vi "Autonomous Independent.vi"   [LabVIEW 2015]
doc: "This VI is called when autonomous begins, and will automatically be terminated when autonomous ends. You can carry out timed or sensor driven robot movement independently without needing to return to the caller."
uses:
  <vilib>/Rock Robotics/WPI/Solenoid/WPI_SolenoidValue.ctl
  <vilib>/Rock Robotics/WPI/Utilities/WPI_GetSetVariantRefNum.vi
  <vilib>/Rock Robotics/Network Tables/NT Read String.vi
  Robot Global Data.vi
  <vilib>/Rock Robotics/WPI/Solenoid/WPI_SolenoidSetEnum.vi
  <vilib>/Rock Robotics/Network Tables/NT Write Numeric Array.vi
panel:
  # "Be sure to right-click and choose Data Operations>>Make Current Value default if you want to save the array values with the VI"
types:
  T1 = typedef "WPI_JoystickDevRef.ctl" = cluster{"Device":T2}
  T2 = typedef "WPI_JoystickDeviceEnum.ctl" = enum16{"USB 0", "USB 1", "USB 2", "USB 3", "USB 4", "USB 5"}
  T3 = typedef "WPI_SolenoidValue.ctl" = enum16{"Off", "On", "Forward", "Reverse"}
  T4 = typedef "WPI_RobotDriveDevRef.ctl" = cluster{"DevStatus":errorcluster, "Motors[]":T5[], "Square Inputs":bool, "Max Output":dbl}
  T5 = typedef "WPI_MotorControlDeviceRef.ctl" = cluster{"DeviceStatus":errorcluster, "Type":T6, "PWM":cluster{"PWM Channel":T7, "DeadBand":T8}, "CAN":cluster{"Device Number":u8, "Control Mode":T9, "Semaphore":T10, "Max Vout":dbl, "TalonSRX Control Mode":T11}, "Invert":bool}
  T6 = typedef "WPI_MotorControlType.ctl" = enum16{"PWM", "CAN", "CANTalonSRX"}
  T7 = typedef "FPGA_DIOPWMChannel.ctl" = enum8{"PWM 0", "PWM 1", "PWM 2", "PWM 3", "PWM 4", "PWM 5", "PWM 6", "PWM 7", "PWM 8", "PWM 9", "PWM MXP 0", "PWM MXP 1", "PWM MXP 2", "PWM MXP 3", "PWM MXP 4", "PWM MXP 5", "PWM MXP 6", "PWM MXP 7", "PWM MXP 8", "PWM MXP 9", "Invalid"}
  T8 = typedef "WPI_PWMDeadband.ctl" = cluster{"Name":string, "maxPositivePwm":i32, "minPositivePwm":i32, "centerPwm":i32, "maxNegativePwm":i32, "minNegativePwm":i32, "angularRange":u16}
  T9 = typedef "WPI_CANJaguar_ControlMode.ctl" = enum8{"Percent VBus", "Current", "Speed", "Position", "Voltage"}
  T10 = typedef "Semaphore RefNum" = refnum<k1>
  T11 = typedef "WPI_CANTalonSRX_APIControlMode.ctl" = enum8{"Percent VBus", "Speed", "Position", "Slave", "Unchanged / Invalid", "Voltage Compensation", "Current", "Motion Profile"}
  T12 = typedef "WPI_SolenoidDevRef.ctl" = cluster{"DevStatus":errorcluster, "Pneumatics Control Module":u8, "Forward Solenoid Channel":T13, "Reverse Solenoid Channel":T13}
  T13 = typedef "WPI_SolenoidChannel.ctl" = enum8{"Solenoid 0", "Solenoid 1", "Solenoid 2", "Solenoid 3", "Solenoid 4", "Solenoid 5", "Solenoid 6", "Solenoid 7", "Invalid"}
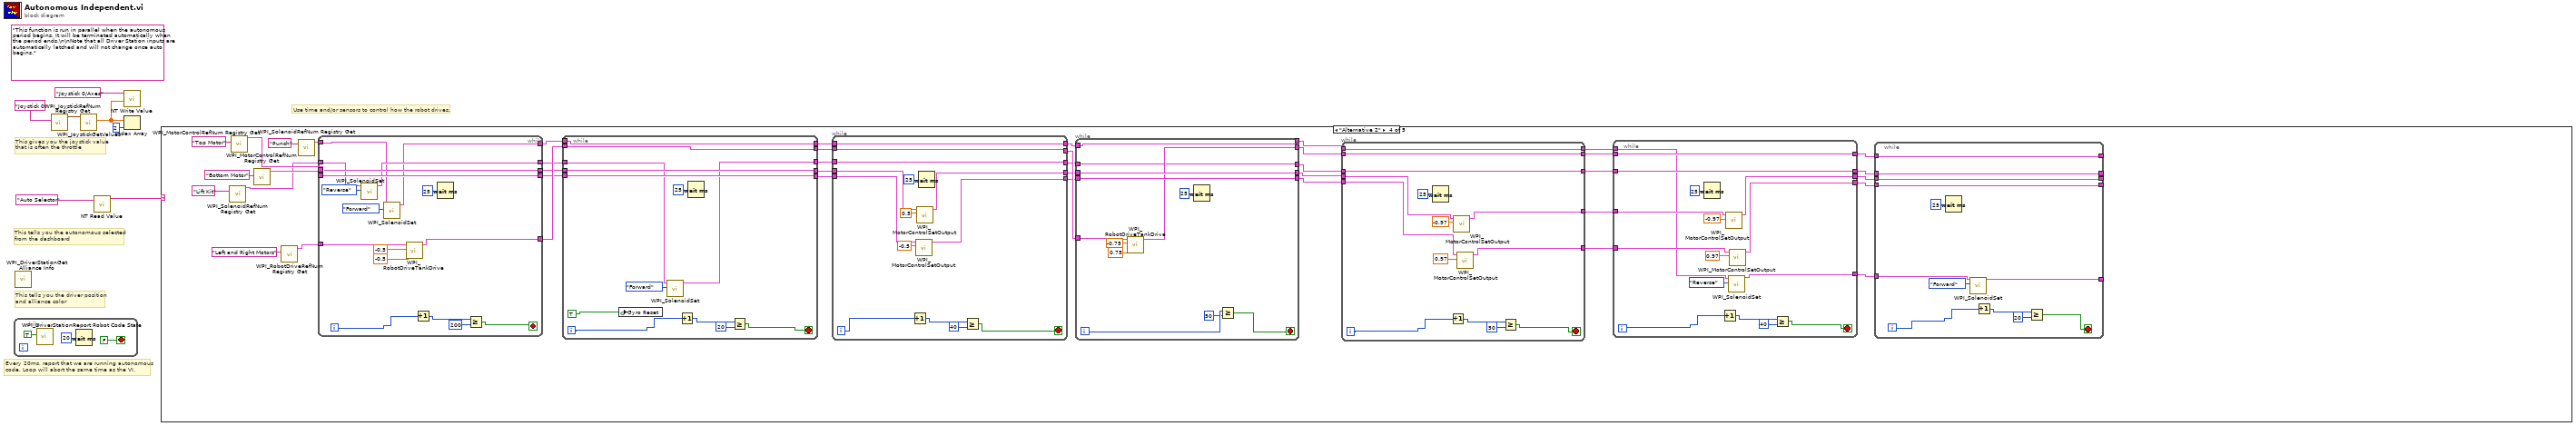
[diagram p0: block diagram]
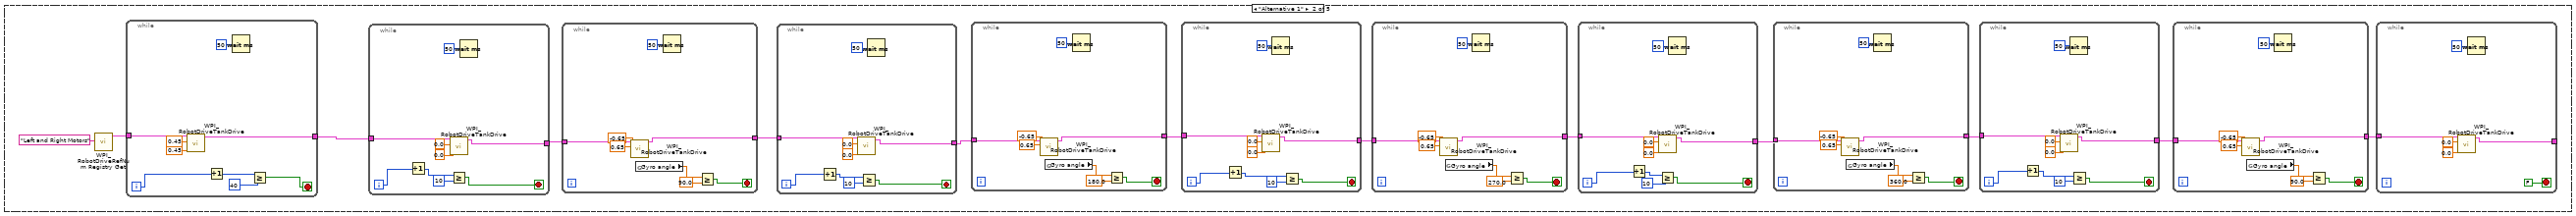
[diagram p3: hidden frame]
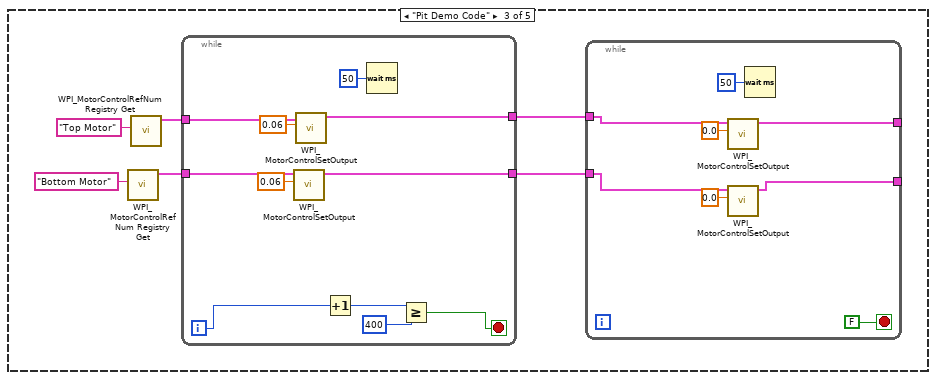
[diagram p4: hidden frame]
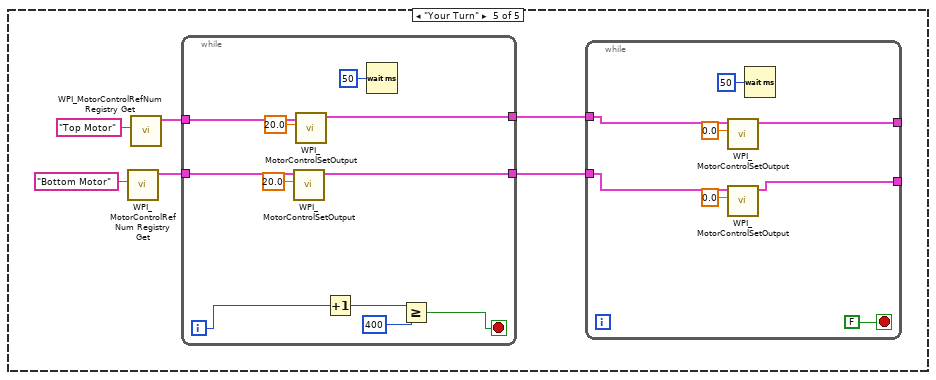
[diagram p5: hidden frame]
diagram:
  (unwired) "This function is run in parallel when the autonomous period begins. It will be terminated automatically when the period ends.\n\nNote that all Driver Station inputs are automatically latched and will not change once auto begins."
  # "This tells you the autonomous selected\nfrom the dashboard"
  # "Every 20ms, report that we are running autonomous\ncode. Loop will abort the same time as the VI."
  # "This gives you the joystick value\nthat is often the throttle"
  # "Use time and/or sensors to control how the robot drives."
  # "This tells you the driver position\nand alliance color"
  n1 = while {
    stop <- FALSE stop-if-true
    n2 = call <vilib>:"WPI_DriverStationReport Robot Code State.vi"("Autonomous"=TRUE) -> ()  [unwired: 10 in, 1 out]
    n3 = Wait (ms)(milliseconds to wait=u32 20) -> ()  [unwired: 1 out]
  }
  n4 = call <vilib>:"WPI_DriverStationGet Alliance Info.vi"() -> ()  [unwired: 12 out]
  n5 = call <vilib>:"WPI_JoystickRefNum Registry Get.vi"("refnum name"="Joystick 0") -> ("JoystickDevRef"=w6:T1)  [unwired: 1 in, 9 out]
  n6 = call <vilib>:"WPI_JoystickGetValues.vi"("JoystickDevRef"=w6) -> ("Axes"=w2:dbl[])  [unwired: 6 in, 4 out]
  n7 = call-poly <vilib>:"NT Read Value.vi"("Name"="Auto Selector") -> ("String"=w3:string)  [unwired: 9 in, 1 out]
  n8 = call-poly <vilib>:"NT Write Value.vi"("Numeric Array"=w2, "Name"="Joystick 0/Axes") -> ()  [unwired: 9 in, 1 out]
  n9 = Index Array(array=w2, index=2) -> ()  [unwired: 1 out]
  n10 = case shown="\"Alternative 2\"" w3 {
    frame Default {
      # "You can put your main auto here, or you can right-click on the case and make any\nother frame be the default case."
      # "This is the frame that will execute if no selection is made, or if it is not recognized"
    }
    frame "Alternative 1" {
      n11 = call <vilib>:"WPI_RobotDriveRefNum Registry Get.vi"("refnum name"="Left and Right Motors") -> ("RobotDriveDevRef"=w23:T4)  [unwired: 9 in, 1 out]
      n12 = while {
        tunnel: w23 -> [w118]
        tunnel: [w117] -> w22
        i -> [w120]
        stop <- w121 stop-if-true
        n13 = call <vilib>:"WPI_RobotDriveTankDrive.vi"("Right axis value"=0.45, "Left axis value"=0.45, "RobotDriveDevRef"=w118) -> ("RobotDriveDevRef"=w117:T4)  [unwired: 6 in, 2 out]
        n14 = Increment(x=w120) -> (x+1=w122:i32)
        n15 = Wait (ms)(milliseconds to wait=u32 50) -> ()  [unwired: 1 out]
        n16 = Greater Or Equal?(x=w122, y=40) -> (x >= y?=w121:bool)
      }
      n17 = while {
        tunnel: w22 -> [w113]
        tunnel: [w110] -> w20
        i -> [w109]
        stop <- w106 stop-if-true
        n18 = Increment(x=w109) -> (x+1=w108:i32)
        n19 = call <vilib>:"WPI_RobotDriveTankDrive.vi"("Right axis value"=0.0, "Left axis value"=0.0, "RobotDriveDevRef"=w113) -> ("RobotDriveDevRef"=w110:T4)  [unwired: 6 in, 2 out]
        n20 = Greater Or Equal?(x=w108, y=10) -> (x >= y?=w106:bool)
        n21 = Wait (ms)(milliseconds to wait=u32 50) -> ()  [unwired: 1 out]
      }
      n22 = while {
        tunnel: w20 -> [w105]
        tunnel: [w98] -> w19
        stop <- w100 stop-if-true
        n23 = call <vilib>:"WPI_RobotDriveTankDrive.vi"("Right axis value"=-0.65, "Left axis value"=0.65, "RobotDriveDevRef"=w105) -> ("RobotDriveDevRef"=w98:T4)  [unwired: 6 in, 2 out]
        n24 = global read "Robot Global Data.vi" "Gyro angle"() -> (w101:dbl)
        n25 = Wait (ms)(milliseconds to wait=u32 50) -> ()  [unwired: 1 out]
        n26 = Greater Or Equal?(x=w101, y=90.0) -> (x >= y?=w100:bool)
      }
      n27 = while {
        tunnel: w19 -> [w96]
        tunnel: [w93] -> w18
        i -> [w92]
        stop <- w89 stop-if-true
        n28 = Increment(x=w92) -> (x+1=w91:i32)
        n29 = call <vilib>:"WPI_RobotDriveTankDrive.vi"("Right axis value"=0.0, "Left axis value"=0.0, "RobotDriveDevRef"=w96) -> ("RobotDriveDevRef"=w93:T4)  [unwired: 6 in, 2 out]
        n30 = Greater Or Equal?(x=w91, y=10) -> (x >= y?=w89:bool)
        n31 = Wait (ms)(milliseconds to wait=u32 50) -> ()  [unwired: 1 out]
      }
      n32 = while {
        tunnel: w18 -> [w88]
        tunnel: [w81] -> w17
        stop <- w83 stop-if-true
        n33 = call <vilib>:"WPI_RobotDriveTankDrive.vi"("Right axis value"=-0.65, "Left axis value"=0.65, "RobotDriveDevRef"=w88) -> ("RobotDriveDevRef"=w81:T4)  [unwired: 6 in, 2 out]
        n34 = global read "Robot Global Data.vi" "Gyro angle"() -> (w84:dbl)
        n35 = Wait (ms)(milliseconds to wait=u32 50) -> ()  [unwired: 1 out]
        n36 = Greater Or Equal?(x=w84, y=180.0) -> (x >= y?=w83:bool)
      }
      n37 = while {
        tunnel: w17 -> [w79]
        tunnel: [w76] -> w16
        i -> [w75]
        stop <- w72 stop-if-true
        n38 = Increment(x=w75) -> (x+1=w74:i32)
        n39 = call <vilib>:"WPI_RobotDriveTankDrive.vi"("Right axis value"=0.0, "Left axis value"=0.0, "RobotDriveDevRef"=w79) -> ("RobotDriveDevRef"=w76:T4)  [unwired: 6 in, 2 out]
        n40 = Wait (ms)(milliseconds to wait=u32 50) -> ()  [unwired: 1 out]
        n41 = Greater Or Equal?(x=w74, y=10) -> (x >= y?=w72:bool)
      }
      n42 = while {
        tunnel: w16 -> [w71]
        tunnel: [w64] -> w15
        stop <- w66 stop-if-true
        n43 = call <vilib>:"WPI_RobotDriveTankDrive.vi"("Right axis value"=-0.65, "Left axis value"=0.65, "RobotDriveDevRef"=w71) -> ("RobotDriveDevRef"=w64:T4)  [unwired: 6 in, 2 out]
        n44 = global read "Robot Global Data.vi" "Gyro angle"() -> (w67:dbl)
        n45 = Wait (ms)(milliseconds to wait=u32 50) -> ()  [unwired: 1 out]
        n46 = Greater Or Equal?(x=w67, y=270.0) -> (x >= y?=w66:bool)
      }
      n47 = while {
        tunnel: w15 -> [w62]
        tunnel: [w59] -> w14
        i -> [w58]
        stop <- w55 stop-if-true
        n48 = Increment(x=w58) -> (x+1=w57:i32)
        n49 = call <vilib>:"WPI_RobotDriveTankDrive.vi"("Right axis value"=0.0, "Left axis value"=0.0, "RobotDriveDevRef"=w62) -> ("RobotDriveDevRef"=w59:T4)  [unwired: 6 in, 2 out]
        n50 = Greater Or Equal?(x=w57, y=10) -> (x >= y?=w55:bool)
        n51 = Wait (ms)(milliseconds to wait=u32 50) -> ()  [unwired: 1 out]
      }
      n52 = while {
        tunnel: w14 -> [w54]
        tunnel: [w47] -> w13
        stop <- w49 stop-if-true
        n53 = call <vilib>:"WPI_RobotDriveTankDrive.vi"("Right axis value"=-0.65, "Left axis value"=0.65, "RobotDriveDevRef"=w54) -> ("RobotDriveDevRef"=w47:T4)  [unwired: 6 in, 2 out]
        n54 = global read "Robot Global Data.vi" "Gyro angle"() -> (w50:dbl)
        n55 = Wait (ms)(milliseconds to wait=u32 50) -> ()  [unwired: 1 out]
        n56 = Greater Or Equal?(x=w50, y=360.0) -> (x >= y?=w49:bool)
      }
      n57 = while {
        tunnel: w13 -> [w45]
        tunnel: [w42] -> w12
        i -> [w41]
        stop <- w38 stop-if-true
        n58 = Increment(x=w41) -> (x+1=w40:i32)
        n59 = call <vilib>:"WPI_RobotDriveTankDrive.vi"("Right axis value"=0.0, "Left axis value"=0.0, "RobotDriveDevRef"=w45) -> ("RobotDriveDevRef"=w42:T4)  [unwired: 6 in, 2 out]
        n60 = Wait (ms)(milliseconds to wait=u32 50) -> ()  [unwired: 1 out]
        n61 = Greater Or Equal?(x=w40, y=10) -> (x >= y?=w38:bool)
      }
      n62 = while {
        tunnel: w12 -> [w37]
        tunnel: [w30] -> w11
        stop <- w32 stop-if-true
        n63 = call <vilib>:"WPI_RobotDriveTankDrive.vi"("Right axis value"=-0.65, "Left axis value"=0.65, "RobotDriveDevRef"=w37) -> ("RobotDriveDevRef"=w30:T4)  [unwired: 6 in, 2 out]
        n64 = global read "Robot Global Data.vi" "Gyro angle"() -> (w33:dbl)
        n65 = Wait (ms)(milliseconds to wait=u32 50) -> ()  [unwired: 1 out]
        n66 = Greater Or Equal?(x=w33, y=90.0) -> (x >= y?=w32:bool)
      }
      n67 = while {
        tunnel: w11 -> [w27]
        tunnel: [w24] -> _
        stop <- FALSE stop-if-true
        n68 = call <vilib>:"WPI_RobotDriveTankDrive.vi"("Right axis value"=0.0, "Left axis value"=0.0, "RobotDriveDevRef"=w27) -> ("RobotDriveDevRef"=w24:T4)  [unwired: 6 in, 2 out]
        n69 = Wait (ms)(milliseconds to wait=u32 50) -> ()  [unwired: 1 out]
      }
    }
    frame "Pit Demo Code" {
      n70 = call <vilib>:"WPI_MotorControlRefNum Registry Get.vi"("refnum name"="Bottom Motor") -> ("MotorControlDevRef"=w129:T5)  [unwired: 9 in, 1 out]
      n71 = call <vilib>:"WPI_MotorControlRefNum Registry Get.vi"("refnum name"="Top Motor") -> ("MotorControlDevRef"=w128:T5)  [unwired: 9 in, 1 out]
      n72 = while {
        tunnel: w129 -> [w148]
        tunnel: w128 -> [w147]
        tunnel: [w141] -> w125
        tunnel: [w140] -> w124
        i -> [w143]
        stop <- w144 stop-if-true
        n73 = call <vilib>:"WPI_MotorControlSetOutput.vi"("Output"=0.06, "MotorControlDevRef"=w148) -> ("MotorControlDevRef"=w140:T5)  [unwired: 7 in, 2 out]
        n74 = call <vilib>:"WPI_MotorControlSetOutput.vi"("Output"=0.06, "MotorControlDevRef"=w147) -> ("MotorControlDevRef"=w141:T5)  [unwired: 7 in, 2 out]
        n75 = Increment(x=w143) -> (x+1=w145:i32)
        n76 = Wait (ms)(milliseconds to wait=u32 50) -> ()  [unwired: 1 out]
        n77 = Greater Or Equal?(x=w145, y=400) -> (x >= y?=w144:bool)
      }
      n78 = while {
        tunnel: w125 -> [w135]
        tunnel: w124 -> [w133]
        tunnel: [w134] -> _
        tunnel: [w132] -> _
        stop <- FALSE stop-if-true
        n79 = call <vilib>:"WPI_MotorControlSetOutput.vi"("Output"=0.0, "MotorControlDevRef"=w135) -> ("MotorControlDevRef"=w134:T5)  [unwired: 7 in, 2 out]
        n80 = call <vilib>:"WPI_MotorControlSetOutput.vi"("Output"=0.0, "MotorControlDevRef"=w133) -> ("MotorControlDevRef"=w132:T5)  [unwired: 7 in, 2 out]
        n81 = Wait (ms)(milliseconds to wait=u32 50) -> ()  [unwired: 1 out]
      }
    }
    frame "Alternative 2" {
      n82 = call <vilib>:"WPI_SolenoidRefNum Registry Get.vi"("refnum name"="Lift Kit") -> ("SolenoidDevRef"=w174:T12)  [unwired: 9 in, 1 out]
      n83 = call <vilib>:"WPI_MotorControlRefNum Registry Get.vi"("refnum name"="Top Motor") -> ("MotorControlDevRef"=w181:T5)  [unwired: 9 in, 1 out]
      n84 = call <vilib>:"WPI_MotorControlRefNum Registry Get.vi"("refnum name"="Bottom Motor") -> ("MotorControlDevRef"=w179:T5)  [unwired: 9 in, 1 out]
      n85 = call <vilib>:"WPI_RobotDriveRefNum Registry Get.vi"("refnum name"="Left and Right Motors") -> ("RobotDriveDevRef"=w185:T4)  [unwired: 9 in, 1 out]
      n86 = call <vilib>:"WPI_SolenoidRefNum Registry Get.vi"("refnum name"="Punch") -> ("SolenoidDevRef"=w171:T12)  [unwired: 9 in, 1 out]
      n87 = while {
        tunnel: w185 -> [w286]
        tunnel: [w279] -> w182
        tunnel: w181 -> [w277]
        tunnel: [w277] -> w180
        tunnel: w179 -> [w276]
        tunnel: [w276] -> w178
        tunnel: w174 -> [w275]
        tunnel: [w274] -> w173
        tunnel: [w270] -> w170
        tunnel: w171 -> [w271]
        i -> [w280]
        stop <- w281 stop-if-true
        n88 = call-poly <vilib>:"WPI_SolenoidSet.vi"("Value"=WPI_SolenoidValue."Reverse", "SolenoidDevRef"=w275) -> ("SolenoidDevRef"=w274:T12)  [unwired: 8 in, 1 out]
        n89 = call-poly <vilib>:"WPI_SolenoidSet.vi"("Value"=WPI_SolenoidValue."Forward", "SolenoidDevRef"=w271) -> ("SolenoidDevRef"=w270:T12)  [unwired: 8 in, 1 out]
        n90 = call <vilib>:"WPI_RobotDriveTankDrive.vi"("Right axis value"=-0.5, "Left axis value"=-0.5, "RobotDriveDevRef"=w286) -> ("RobotDriveDevRef"=w279:T4)  [unwired: 6 in, 2 out]
        n91 = Increment(x=w280) -> (x+1=w283:i32)
        n92 = Wait (ms)(milliseconds to wait=u32 25) -> ()  [unwired: 1 out]
        n93 = Greater Or Equal?(x=w283, y=200) -> (x >= y?=w281:bool)
      }
      n94 = while {
        tunnel: [w227] -> w158
        tunnel: w182 -> [w227]
        tunnel: [w220] -> w154
        tunnel: w180 -> [w220]
        tunnel: [w219] -> w153
        tunnel: w178 -> [w219]
        tunnel: w173 -> [w217]
        tunnel: [w216] -> w152
        tunnel: w170 -> [w215]
        tunnel: [w215] -> w156
        i -> [w222]
        stop <- w223 stop-if-true
        n95 = global write "Robot Global Data.vi" "Gyro Reset"(TRUE) -> ()
        n96 = call-poly <vilib>:"WPI_SolenoidSet.vi"("Value"=WPI_SolenoidValue."Forward", "SolenoidDevRef"=w217) -> ("SolenoidDevRef"=w216:T12)  [unwired: 8 in, 1 out]
        n97 = Increment(x=w222) -> (x+1=w224:i32)
        n98 = Wait (ms)(milliseconds to wait=u32 25) -> ()  [unwired: 1 out]
        n99 = Greater Or Equal?(x=w224, y=20) -> (x >= y?=w223:bool)
      }
      n100 = while {
        tunnel: [w202] -> w157
        tunnel: w158 -> [w202]
        tunnel: [w201] -> w155
        tunnel: w156 -> [w201]
        tunnel: w154 -> [w200]
        tunnel: w153 -> [w199]
        tunnel: [w196] -> w151
        tunnel: w152 -> [w196]
        tunnel: [w195] -> w150
        tunnel: [w194] -> w149
        i -> [w190]
        stop <- w189 stop-if-true
        n101 = Increment(x=w190) -> (x+1=w192:i32)
        n102 = call <vilib>:"WPI_MotorControlSetOutput.vi"("Output"=-0.5, "MotorControlDevRef"=w199) -> ("MotorControlDevRef"=w194:T5)  [unwired: 7 in, 2 out]
        n103 = call <vilib>:"WPI_MotorControlSetOutput.vi"("Output"=0.5, "MotorControlDevRef"=w200) -> ("MotorControlDevRef"=w195:T5)  [unwired: 7 in, 2 out]
        n104 = Wait (ms)(milliseconds to wait=u32 25) -> ()  [unwired: 1 out]
        n105 = Greater Or Equal?(x=w192, y=40) -> (x >= y?=w189:bool)
      }
      n106 = while {
        tunnel: w157 -> [w269]
        tunnel: w150 -> [w265]
        tunnel: [w265] -> w160
        tunnel: [w264] -> w159
        tunnel: w149 -> [w264]
        tunnel: [w263] -> w162
        tunnel: [w262] -> w161
        tunnel: w151 -> [w262]
        tunnel: [w261] -> w163
        tunnel: w155 -> [w261]
        i -> [w260]
        stop <- w259 stop-if-true
        n107 = call <vilib>:"WPI_RobotDriveTankDrive.vi"("Right axis value"=0.75, "Left axis value"=-0.75, "RobotDriveDevRef"=w269) -> ("RobotDriveDevRef"=w263:T4)  [unwired: 6 in, 2 out]
        n108 = Wait (ms)(milliseconds to wait=u32 25) -> ()  [unwired: 1 out]
        n109 = Greater Or Equal?(x=w260, y=50) -> (x >= y?=w259:bool)
      }
      n110 = while {
        tunnel: [w250] -> w184
        tunnel: [w249] -> w183
        tunnel: w160 -> [w248]
        tunnel: w159 -> [w247]
        tunnel: [w246] -> w177
        tunnel: w162 -> [w246]
        tunnel: [w245] -> w172
        tunnel: w161 -> [w245]
        tunnel: w163 -> [w244]
        tunnel: [w244] -> w169
        i -> [w251]
        stop <- w252 stop-if-true
        n111 = Wait (ms)(milliseconds to wait=u32 25) -> ()  [unwired: 1 out]
        n112 = Increment(x=w251) -> (x+1=w254:i32)
        n113 = call <vilib>:"WPI_MotorControlSetOutput.vi"("Output"=-0.97, "MotorControlDevRef"=w248) -> ("MotorControlDevRef"=w250:T5)  [unwired: 7 in, 2 out]
        n114 = call <vilib>:"WPI_MotorControlSetOutput.vi"("Output"=0.97, "MotorControlDevRef"=w247) -> ("MotorControlDevRef"=w249:T5)  [unwired: 7 in, 2 out]
        n115 = Greater Or Equal?(x=w254, y=50) -> (x >= y?=w252:bool)
      }
      n116 = while {
        tunnel: w184 -> [w236]
        tunnel: w183 -> [w235]
        tunnel: [w233] -> w164
        tunnel: w177 -> [w233]
        tunnel: [w232] -> w165
        tunnel: w172 -> [w232]
        tunnel: w169 -> [w231]
        tunnel: [w230] -> w168
        tunnel: [w229] -> w166
        tunnel: [w228] -> w167
        i -> [w237]
        stop <- w238 stop-if-true
        n117 = Wait (ms)(milliseconds to wait=u32 25) -> ()  [unwired: 1 out]
        n118 = Increment(x=w237) -> (x+1=w240:i32)
        n119 = call <vilib>:"WPI_MotorControlSetOutput.vi"("Output"=-0.97, "MotorControlDevRef"=w236) -> ("MotorControlDevRef"=w229:T5)  [unwired: 7 in, 2 out]
        n120 = call-poly <vilib>:"WPI_SolenoidSet.vi"("Value"=WPI_SolenoidValue."Reverse", "SolenoidDevRef"=w231) -> ("SolenoidDevRef"=w230:T12)  [unwired: 8 in, 1 out]
        n121 = call <vilib>:"WPI_MotorControlSetOutput.vi"("Output"=0.97, "MotorControlDevRef"=w235) -> ("MotorControlDevRef"=w228:T5)  [unwired: 7 in, 2 out]
        n122 = Greater Or Equal?(x=w240, y=40) -> (x >= y?=w238:bool)
      }
      n123 = while {
        tunnel: w168 -> [w212]
        tunnel: w167 -> [w211]
        tunnel: w166 -> [w208]
        tunnel: w165 -> [w209]
        tunnel: w164 -> [w210]
        tunnel: [w211] -> _
        tunnel: [w210] -> _
        tunnel: [w209] -> _
        tunnel: [w208] -> _
        tunnel: [w207] -> _
        i -> [w203]
        stop <- w204 stop-if-true
        n124 = Wait (ms)(milliseconds to wait=u32 25) -> ()  [unwired: 1 out]
        n125 = call-poly <vilib>:"WPI_SolenoidSet.vi"("Value"=WPI_SolenoidValue."Forward", "SolenoidDevRef"=w212) -> ("SolenoidDevRef"=w207:T12)  [unwired: 8 in, 1 out]
        n126 = Increment(x=w203) -> (x+1=w205:i32)
        n127 = Greater Or Equal?(x=w205, y=20) -> (x >= y?=w204:bool)
      }
    }
    frame "Your Turn" {
      n128 = call <vilib>:"WPI_MotorControlRefNum Registry Get.vi"("refnum name"="Bottom Motor") -> ("MotorControlDevRef"=w292:T5)  [unwired: 9 in, 1 out]
      n129 = call <vilib>:"WPI_MotorControlRefNum Registry Get.vi"("refnum name"="Top Motor") -> ("MotorControlDevRef"=w291:T5)  [unwired: 9 in, 1 out]
      n130 = while {
        tunnel: w292 -> [w311]
        tunnel: w291 -> [w310]
        tunnel: [w304] -> w288
        tunnel: [w303] -> w287
        i -> [w306]
        stop <- w307 stop-if-true
        n131 = call <vilib>:"WPI_MotorControlSetOutput.vi"("Output"=20.0, "MotorControlDevRef"=w311) -> ("MotorControlDevRef"=w303:T5)  [unwired: 7 in, 2 out]
        n132 = call <vilib>:"WPI_MotorControlSetOutput.vi"("Output"=20.0, "MotorControlDevRef"=w310) -> ("MotorControlDevRef"=w304:T5)  [unwired: 7 in, 2 out]
        n133 = Increment(x=w306) -> (x+1=w308:i32)
        n134 = Wait (ms)(milliseconds to wait=u32 50) -> ()  [unwired: 1 out]
        n135 = Greater Or Equal?(x=w308, y=400) -> (x >= y?=w307:bool)
      }
      n136 = while {
        tunnel: w288 -> [w298]
        tunnel: w287 -> [w296]
        tunnel: [w297] -> _
        tunnel: [w295] -> _
        stop <- FALSE stop-if-true
        n137 = call <vilib>:"WPI_MotorControlSetOutput.vi"("Output"=0.0, "MotorControlDevRef"=w298) -> ("MotorControlDevRef"=w297:T5)  [unwired: 7 in, 2 out]
        n138 = call <vilib>:"WPI_MotorControlSetOutput.vi"("Output"=0.0, "MotorControlDevRef"=w296) -> ("MotorControlDevRef"=w295:T5)  [unwired: 7 in, 2 out]
        n139 = Wait (ms)(milliseconds to wait=u32 50) -> ()  [unwired: 1 out]
      }
    }
  }
